vi "UpdateDropletTable.vi"(8 "error in (no error)":errorcluster) -> (0 "error out":errorcluster, 3 "DropletTabeVariant":variant)   [LabVIEW 2013]
doc: "Use this template to build a VI to use as a subVI."
uses:
  DB/DbEnum.ctl
  DB/DropletDB.ctl
  TypeDef/DropletDisplay.ctl
  <vilib>/vision/Image Controls.llb/IMAQ Image.ctl
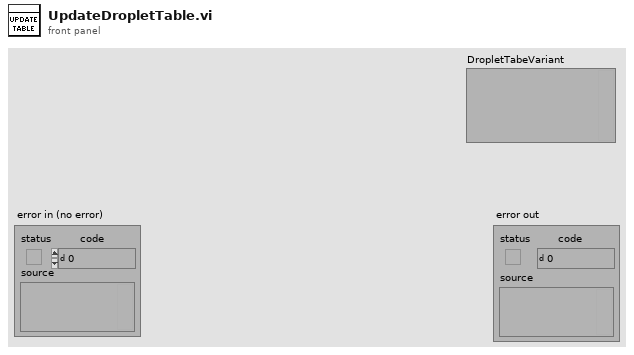
[diagram p1: front panel]
types:
  T1 = typedef "DropletDB.ctl" = cluster{"ImageFreezeIndex":i32, "DropIndex":i32, "Position":cluster{"x":sgl, "y":sgl}, "Bounding Box":cluster{"x":sgl, "y":sgl}[], "Score":sgl, "GreyLevelInBoundingBox":dbl[], "GLDifference":dbl[], "Baseline level":dbl, "Peak":cluster{"Value":dbl, "Index":u32}, "Peak Onset":cluster{"Value":dbl, "Index":u32}, "FreezeFileName":string, "FreezeAbsTime":timestamp, "FreezeTemperature":dbl, "ImageIndexArray":u32[], "Freeze Point Found":bool, "Baseline std":dbl, "FreezedImageArray":cluster{"Image":u8[][]}[], "Include Droplet":bool, "Remark":string, "Freeze Rel Time":u32[], "Diameter (microns)":dbl}[]
  T2 = typedef "DbEnum.ctl" = enum16{"Write DropletDB", "Init", "Insert Detection Result Data", "Insert Grey Level Result", "Insert Baseline Results", "AddFreezeImagesAtCertainDroplet", "UpdateIncludeDroplet", "Insert Freeze Analysis Results", "GetDropDB", "GetNoFreezedDroplets", "GetGreyLevelAndDiff", "GetGreyLevelatIndexTime", "GetDropletsBoundingBox", "GetDropletsDiameter"}
  T3 = typedef "DropletDisplay.ctl" = cluster{"Drop Info":dbl[], "Freeze Images":T4[], "Include Droplet":bool, "Remark":string}[]
  T4 = typedef "IMAQ Image.ctl" = refnum<image>
  T5 = cluster{"Drop Info":dbl[], "Freeze Images":T4[], "Include Droplet":bool, "Remark":string}
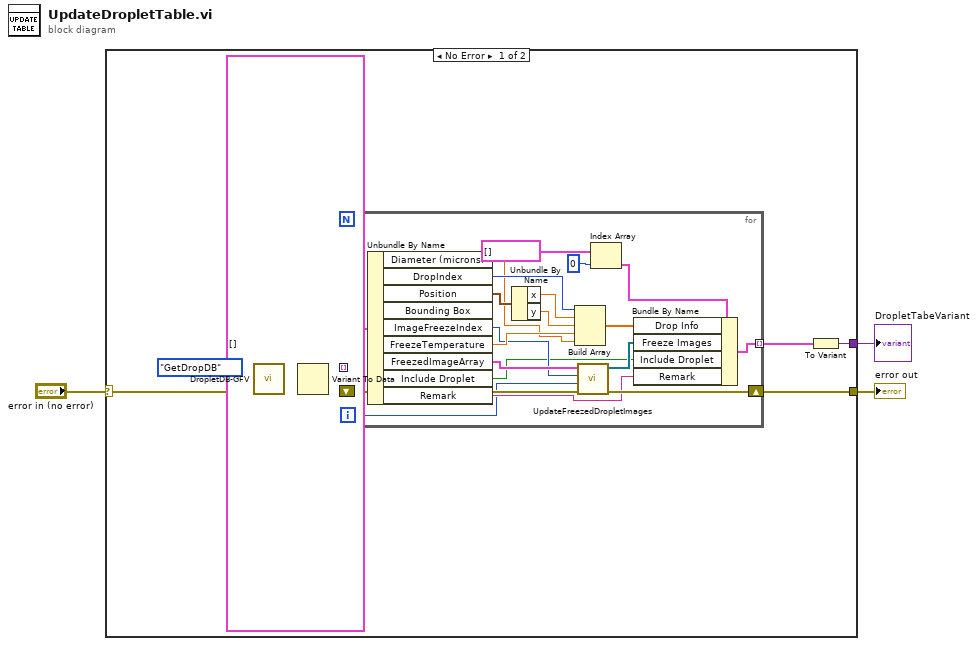
[diagram p0: block diagram]
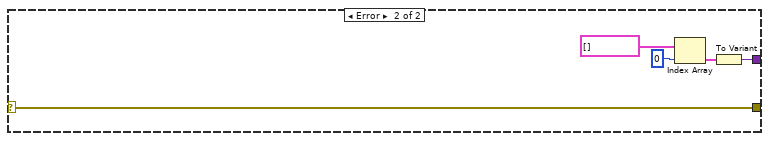
[diagram p2: hidden frame]
diagram:
  n1 = case shown="No Error" "error in (no error)" {
    selector: "error in (no error)" -> [w5 w38]
    tunnel: [w8 w38] -> w2
    tunnel: [w6 w35] -> w1
    frame No Error {
      n2 = call "DropletDB-GFV.vi"("error in (no error)"=w5, "Command In"=DbEnum."GetDropDB") -> ("error out"=w12:errorcluster, "Data out"=w13:variant)  [unwired: 8 in]
      n3 = Variant To Data(error in=w12, type=T1 [] ("DropletArray"), Variant=w13) -> (data=w10:T1, error out=w4:errorcluster)
      n4 = for {
        tunnel: w10 -> [w33] mode=indexing
        shift-right: [w21] -> w8
        shift-left: w4 -> [w22]
        tunnel: [w29] -> w7 mode=indexing
        i -> [w15]
        n5 = Unbundle By Name(w33) -> ("Diameter (microns)"=w14:dbl, "DropIndex"=w23:i32, "Position"=w28:cluster{"x":sgl, "y":sgl}, "ImageFreezeIndex"=w19:i32, "FreezeTemperature"=w25:dbl, "FreezedImageArray"=w20:cluster{"Image":u8[][]}[], "Include Droplet"=w17:bool, "Remark"=w16:string)  [unwired: 1 out]
        n6 = Unbundle By Name(w28) -> ("x"=w27:sgl, "y"=w26:sgl)
        n7 = Build Array(w23, w27, w26, w25, w14) -> (w24:dbl[])
        n8 = call "UpdateFreezedDropletImages.vi"("error in (no error)"=w22, "DropletNumber"=w15, "FreezeRelTime(sec)"=w19, "FreezedImageArray"=w20) -> ("error out"=w21:errorcluster, "OutputFreezedImagesRef"=w18:T4[])  [unwired: 6 in]
        n9 = Index Array(array=T3 [] ("Droplet Display"), index=0) -> (element=w30:T5)
        n10 = Bundle By Name(cluster=w30, "Drop Info"=w24, "Freeze Images"=w18, "Include Droplet"=w17, "Remark"=w16) -> (w29:T5)
      }
      n11 = To Variant(anything=w7) -> (Variant=w6:variant)
    }
    frame Error {
      n12 = Index Array(array=T3 [] ("Droplet Display"), index=0) -> (element=w34:T5)
      n13 = To Variant(anything=w34) -> (Variant=w35:variant)
    }
  }
  "error out" <- w2
  "DropletTabeVariant" <- w1
